vi "KE622x -- Clear Trace Buffer.vi"(0 "Resource In":refnum<visa-resource-name>, 1 "Check For SCPI Errors? (T)":bool=TRUE, 11 "error in (no error)":errorcluster) -> (4 "Resource Out (dupl)":refnum<visa-resource-name>, 15 "error out":errorcluster)   [LabVIEW 2019, in "Keithley 622x.lvlib"]
uses:
  Keithley 622x.lvlib
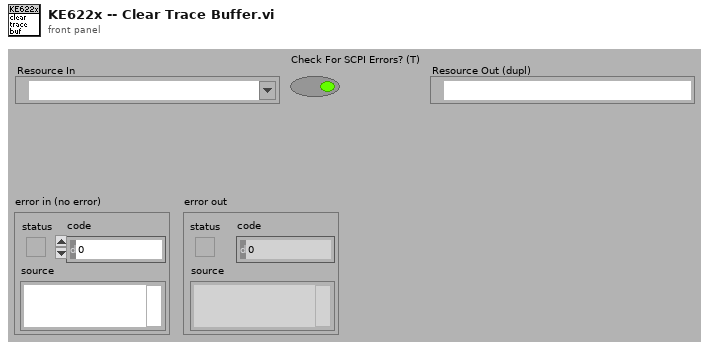
[diagram p1: front panel]
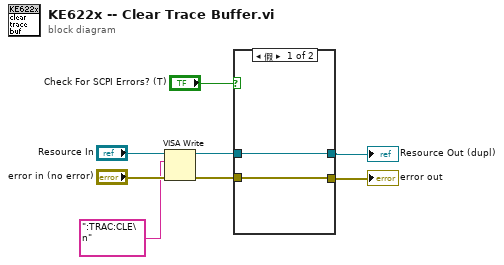
[diagram p0: block diagram]
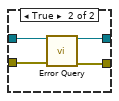
[diagram p2: hidden frame]
diagram:
  n1 = VISA Write(VISA resource name="Resource In", write buffer=":TRAC:CLE\n" ("format string"), error in (no error)="error in (no error)") -> (VISA resource name out=w5:refnum<visa-resource-name>, error out=w4:errorcluster)  [unwired: 1 out]
  n2 = case shown="假" "Check For SCPI Errors? (T)" {
    tunnel: w5 -> [w10 w14]
    tunnel: w4 -> [w9 w13]
    tunnel: [w9 w12] -> w1
    tunnel: [w10 w11] -> w2
    frame False {
    }
    frame True {
      n3 = call "Error Query.vi"("VISA Resource In"=w14, "error in (no error)"=w13) -> ("VISA Resource Out (dupl)"=w11:refnum<visa-resource-name>, "error out"=w12:errorcluster)  [unwired: 10 in, 2 out]
    }
  }
  "Resource Out (dupl)" <- w2
  "error out" <- w1
